vi "encodeStream.vi"(8 "error in (no error)":errorcluster, 11 "tBSONString in":refnum<class "tBSONString.lvclass">) -> (0 "error out":errorcluster, 2 "Byte Array":u8[](array[numeric]), 3 "tBSONString out":refnum<class "tBSONString.lvclass">)   [LabVIEW 2013, in "BSON.lvlib" / "tBSONString.lvclass"]
uses:
  tBSONString.lvclass
  tBSONElement/tBSONElement.lvclass
  getValue.vi
  BSON.lvlib
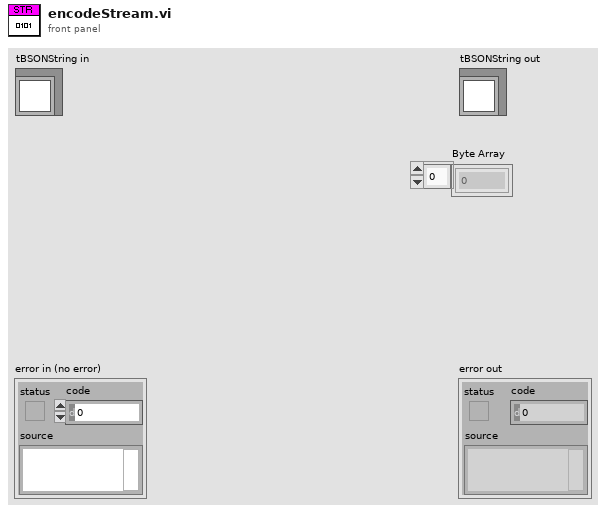
[diagram p1: front panel]
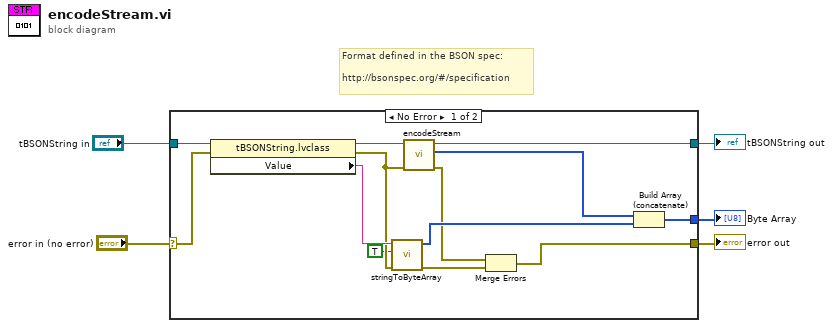
[diagram p0: block diagram]
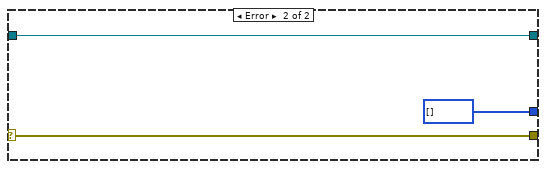
[diagram p2: hidden frame]
diagram:
  # "Format defined in the BSON spec:\n\nhttp://bsonspec.org/#/specification"
  n1 = case shown="No Error" "error in (no error)" {
    selector: "error in (no error)" -> [w17 w20]
    tunnel: "tBSONString in" -> [w18 w21]
    tunnel: [w11 w21] -> w3
    tunnel: [w6 w20] -> w2
    tunnel: [w16 u8[] []] -> w1
    frame No Error {
      n2 = property class="tBSONString.lvclass"(reference=w18, error in=w17) -> (reference out=w12:refnum<class "tBSONString.lvclass">, error out=w10:errorcluster, "Value"=w15:string)
      n3 = call "stringToByteArray.vi"("error in (no error)"=w10, "Prepend Size"=TRUE, "String"=w15) -> ("error out"=w14:errorcluster, "byte array"=w13:u8[])  [unwired: 7 in]
      n4 = call-parent "encodeStream.vi"("error in (no error)"=w10, "tBSONElement in"=w12) -> ("error out"=w9:errorcluster, "Byte Array"=w8:u8[], "tBSONElement out"=w11:refnum<class "tBSONString.lvclass">)  [unwired: 7 in]
      n5 = Merge Errors(w9, w14) -> (w6:errorcluster)
      n6 = Build Array (concatenate)(w8, w13) -> (w16:u8[])
    }
    frame Error {
    }
  }
  "error out" <- w2
  "tBSONString out" <- w3
  "Byte Array" <- w1
